vi "02-sqrt_with_error_processing.vi"() -> ()   [LabVIEW 2018, in "LV-0mq-Julia_roundtrip-lib.lvlib"]
uses:
  LV-0mq-Julia_roundtrip-lib.lvlib
  Server or client state.ctl
  detailed error info.ctl
  StackFrame.ctl
  Commands.ctl
  f447f3f0-0a94-48e6-8be8-e8543bd34c86.vi
  f447f3f0-0a94-48e6-8be8-e8543bd34c86.vi/e03cbec3-9004-442f-8b1d-848ee65d7d82.vi
  f447f3f0-0a94-48e6-8be8-e8543bd34c86.vi/e03cbec3-9004-442f-8b1d-848ee65d7d82.vi/b611a249-1f85-403a-a17e-30a6252b92d1.vi
  f447f3f0-0a94-48e6-8be8-e8543bd34c86.vi/e03cbec3-9004-442f-8b1d-848ee65d7d82.vi/a245c890-0bba-4eb6-9978-6db9adda47c5.vi
  f447f3f0-0a94-48e6-8be8-e8543bd34c86.vi/e03cbec3-9004-442f-8b1d-848ee65d7d82.vi/ea1158ea-257a-4be6-a021-317dd3546ac9.vi
  jl-scripts path.vi
  check ID validity.vi
  bindata_descr to JSON.vi
  check cluster field names.vi
  concat JSON.vi
  call Jl server fn.vi
  jl stack traces global.vi
panel:
  in  "x":dbl=2.0
  in  "next":bool
  out "sqrt":dbl=nan
  out "detailed error info":T1
  out "current error":errorcluster
  out "final error":errorcluster
  out "short err code":u8
  in  "stop":bool
  out "ZMQ timeout":bool
  out "Julia script file path":path
  out "temporary script path":path
  out "Jl Server state":T3
  # "On a negative argument, an exception occurs in Julia. \n\nThe Julia server catches the exception and passes the information to the LV client:  Below you get detailed error information.\n\nFurthermore, the last 1024 (you can change the number) exceptions in the current session are logged into the global \"jl stack traces global.vi\".  On exception, this VI opens the front panel of that global."
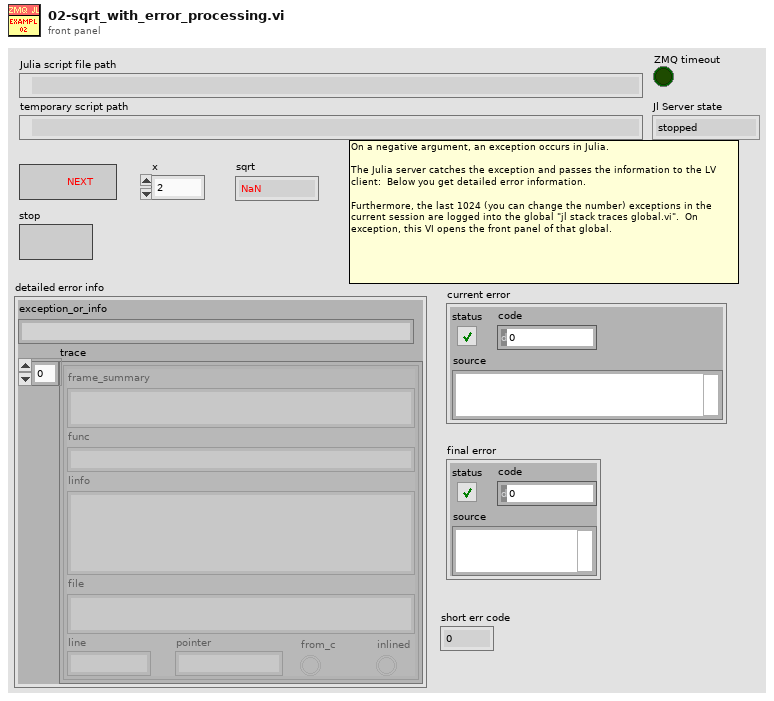
[diagram p1: front panel]
types:
  T1 = typedef "LV-0mq-Julia_roundtrip-lib.lvlib/detailed error info.ctl" = cluster{"exception_or_info":string, "trace":T2[]}
  T2 = typedef "LV-0mq-Julia_roundtrip-lib.lvlib/StackFrame.ctl" = cluster{"frame_summary":string, "func":string, "linfo":string, "file":string, "line":i32, "pointer":u64, "from_c":bool, "inlined":bool}
  T3 = typedef "LV-0mq-Julia_roundtrip-lib.lvlib/Server or client state.ctl" = enum16{"stopped", "running", "unknown"}
  T4 = typedef "LV-0mq-Julia_roundtrip-lib.lvlib/Commands.ctl" = enum16{"Start Jl-server & Init LV-client", "Send request & Get response ", "Stop Jl-server & Cleanup LV-client", "Cleanup LV-client", "Start Jl-server", "Stop Jl-server", "Init LV-Client", "Cleanup LV-Client", "(not allowed)", "Set LV Client state", "Set Jl Server state", "set ZMQ timeout", "read ZMQ timeout", "read-out state"}
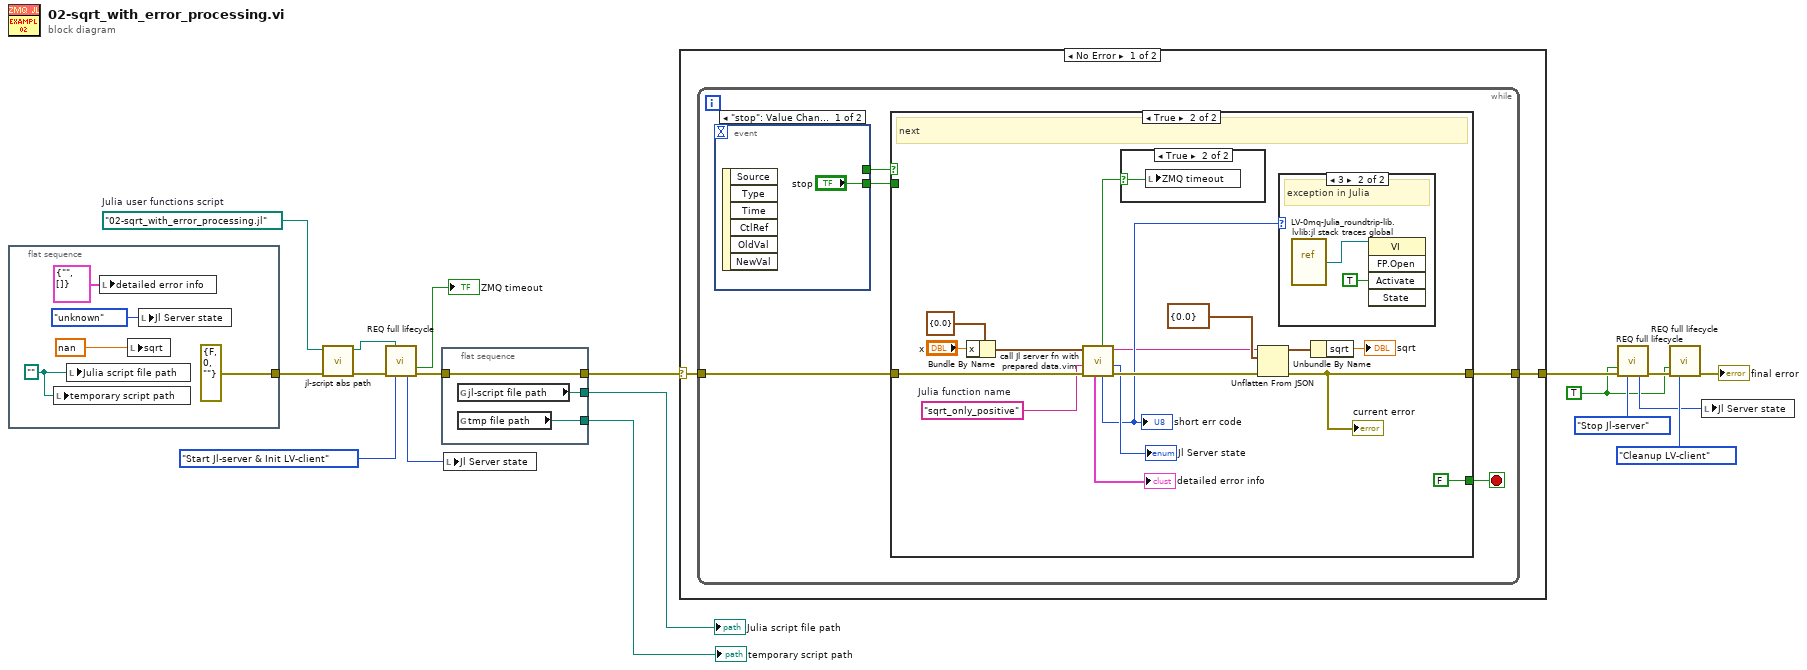
[diagram p0: block diagram]
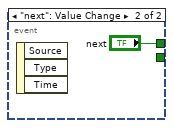
[diagram p2: hidden frame]
diagram:
  w4 = path "02-sqrt_with_error_processing.jl"  # Julia user functions script
  w1 = TRUE ("Force command")
  n1 = flat-sequence {
    tunnel: [errorcluster {"status"=FALSE, "code"=0, "source"=""} ("error in (no error)")] -> w2
    frame #0 {
      w19 = path ""
      n2 = local write "temporary script path"(w19) -> ()
      n3 = local write "Julia script file path"(w19) -> ()
      n4 = local write "detailed error info"(T1 {"exception_or_info"="", "trace"=[]} ("detailed error info")) -> ()
      n5 = local write "sqrt"(nan ("Server response")) -> ()
      n6 = local write "Jl Server state"(Server_or_client_state."unknown" ("Jl Server state out")) -> ()
    }
  }
  n7 = call "jl-script abs path.vi"("error in (no error)"=w2, "Julia user functions script"=w4) -> ("error out"=w5:errorcluster, "script abs path"=w6:path)  [unwired: 8 in]
  n8 = call "REQ full lifecycle.vi"("Julia user functions script"=w6, "error in"=w5, "command"=Commands."Start Jl-server & Init LV-client") -> ("timeout?"=→"ZMQ timeout":bool, "Jl Server state out"=w8:T3, "error out"=w7:errorcluster)  [unwired: 6 in, 4 out]
  n9 = flat-sequence {
    tunnel: [w26] -> w13
    tunnel: w7 -> [w26]
    tunnel: [w25] -> w11
    tunnel: [w24] -> w12
    frame #0 {
      n10 = global read "jl-scripts path.vi" "jl-script file path"() -> (w25:path)
      n11 = global read "jl-scripts path.vi" "tmp file path"() -> (w24:path)
    }
  }
  n12 = local write "Jl Server state"(w8) -> ()
  n13 = case shown="No Error" w13 {
    selector: w13 -> [w27 w57]
    tunnel: [w28 w57] -> w18
    frame No Error {
      n14 = while {
        tunnel: w27 -> [w32]
        tunnel: [w33] -> w28
        stop <- w30 stop-if-true
        n15 = event shown="[0] \"stop\": Value Change" {
          selector: _ -> [_ _]
          dyn-events: _ -> [_ _]
          timeout: _ -> [_ _]
          tunnel: [_ "next"] -> w31
          tunnel: ["stop" _] -> w29
          event "stop": Value Change {
            n16 = event-data() -> ()  [unwired: 1 in, 6 out]
          }
          event "next": Value Change {
            n17 = event-data() -> ()  [unwired: 1 in, 3 out]
          }
        }
        n18 = case shown="True" w31 {
          tunnel: [w37 w50] -> w33
          tunnel: w32 -> [w37 w45]
          tunnel: [w36 FALSE ("stop this VI only")] -> w30
          tunnel: w29 -> [w36 _]
          frame False {
            # "stop"
          }
          frame True {
            w44 = "sqrt_only_positive"  # Julia function name
            # "next"
            n19 = Bundle By Name(cluster=cluster{"x":dbl} {"x"=0.0}, "x"="x") -> (w43:cluster{"x":dbl})
            n20 = call "call Jl server fn with prepared data.vim"("error in (no error)"=w45, "fun2call"=w44, "Arguments 1"=w43) -> ("error out"=w46:errorcluster, "Jl Server state out"=→"Jl Server state":T3, "JSON received"=w38:string, "return code"=w39:u8, "timeout?"=w40:bool, "detailed error info"=→"detailed error info":T1)  [unwired: 2 in, 1 out]
            "short err code" <- w39
            n21 = case shown="True" w40 {
              selector: w40 -> [_ w56]
              frame False {
              }
              frame True {
                n22 = local write "ZMQ timeout"(w56) -> ()
              }
            }
            n23 = Unflatten From JSON(JSON string=w38, type and defaults=cluster{"sqrt":dbl} {"sqrt"=0.0} ("parsed response"), error in (no error)=w46) -> (value=w52:cluster{"sqrt":dbl}, error out=w50:errorcluster)  [unwired: 4 in]
            "current error" <- w50
            n24 = case shown="3" w39 {
              frame 0, Default {
              }
              frame 3 {
                # "exception in Julia"
                n25 = vi-ref "LV-0mq-Julia_roundtrip-lib.lvlib:jl stack traces global.vi"() -> (w54:refnum<vi>)
                n26 = invoke class="VI" method="FP.Open"(reference=w54, "Activate"=TRUE ("Activate?")) -> ()  [unwired: 3 in, 5 out]
              }
            }
            n27 = Unbundle By Name(w52) -> ("sqrt"=→"sqrt":dbl)
          }
        }
      }
    }
    frame Error {
    }
  }
  n28 = call "REQ full lifecycle.vi"("Force command"=w1, "error in"=w18, "command"=Commands."Stop Jl-server") -> ("Jl Server state out"=w10:T3, "error out"=w16:errorcluster)  [unwired: 6 in, 5 out]
  n29 = call "REQ full lifecycle.vi"("Force command"=w1, "error in"=w16, "command"=Commands."Cleanup LV-client") -> ("error out"=→"final error":errorcluster)  [unwired: 6 in, 6 out]
  n30 = local write "Jl Server state"(w10) -> ()
  "temporary script path" <- w12
  "Julia script file path" <- w11
